vi "Read Size.vi"(8 "error in (no error)":errorcluster, 11 "UIStep in":refnum<class "UIStep.lvclass">) -> (0 "error out":errorcluster, 2 "Size":enum16{"Small", "Middle", "Big"}(ring), 3 "UIStep out":refnum<class "UIStep.lvclass">)   [LabVIEW 2015, in "UIStep.lvclass"]
uses:
  UIStep.lvclass
  UIStep.lvclass/UIStep.ctl
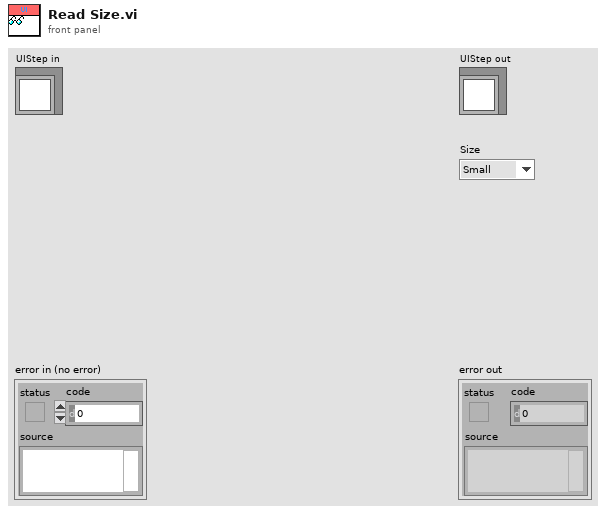
[diagram p1: front panel]
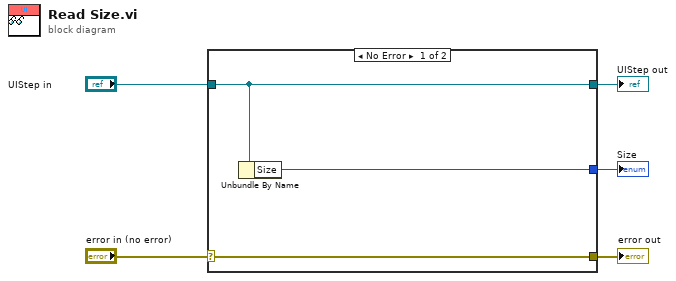
[diagram p0: block diagram]
diagram:
  n1 = case shown="No Error" "error in (no error)" {
    selector: "error in (no error)" -> [w8 w9]
    tunnel: [w8 w9] -> w4
    tunnel: [w7 w10] -> w2
    tunnel: "UIStep in" -> [w7 w10]
    tunnel: [w6 _] -> w1
    frame No Error {
      n2 = Unbundle By Name(w7) -> ("Size"=w6:enum16{"Small", "Middle", "Big"})
    }
    frame Error {
    }
  }
  "error out" <- w4
  "UIStep out" <- w2
  "Size" <- w1
